vi "5010 Image Sizes Not Equal.vi"(8 "error in (no error)":errorcluster) -> (0 "error out":errorcluster)   [LabVIEW 2020, in "MacroAssert.lvlib" / "Custom Errors.lvlib"]
uses:
  Custom Errors.lvlib
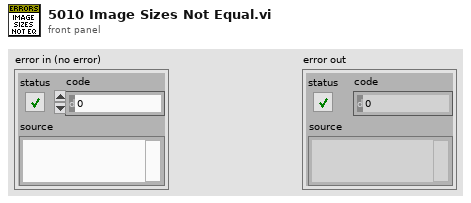
[diagram p1: front panel]
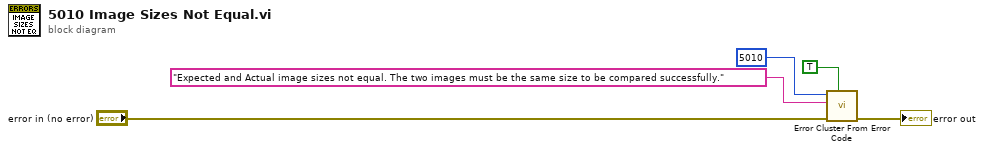
[diagram p0: block diagram]
diagram:
  n1 = call <vilib>:"Error Cluster From Error Code.vi"("show call chain? (False)"=TRUE, "error in (no error)"="error in (no error)", "error message (\"\")"="Expected and Actual image sizes not equal. The two images must be the same size to be compared successfully.", "error code (0)"=5010) -> ("error out"=→"error out":errorcluster)  [unwired: 5 in]
